vi "Untitled 2.vi"(8 "shift":i8, 10 "number":u16) -> (0 "newNumber":u16, 3 "isOdd?":bool)   [LabVIEW 2016]
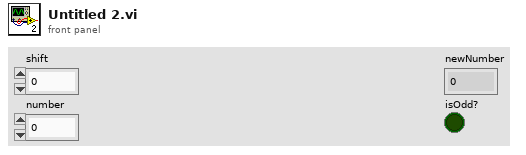
[diagram p1: front panel]
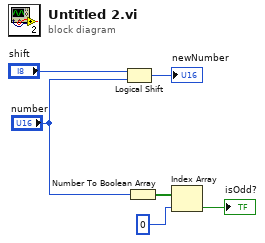
[diagram p0: block diagram]
diagram:
  n1 = Logical Shift(y="shift", x="number") -> (x << y=→"newNumber":u16)
  n2 = Number To Boolean Array(number="number") -> (Boolean array=w3:bool[])
  n3 = Index Array(array=w3, index=0) -> (element=→"isOdd?":bool)
